vi "Benchmarks_DVR.vi"() -> ()   [LabVIEW 2024]
uses:
  <vilib>/numeric/Random Number (Range) U64.vi
  <vilib>/numeric/sub_Random U32.vi
panel:
  out "Waveform Chart":dbl(graph)
  out "Numeric":dbl
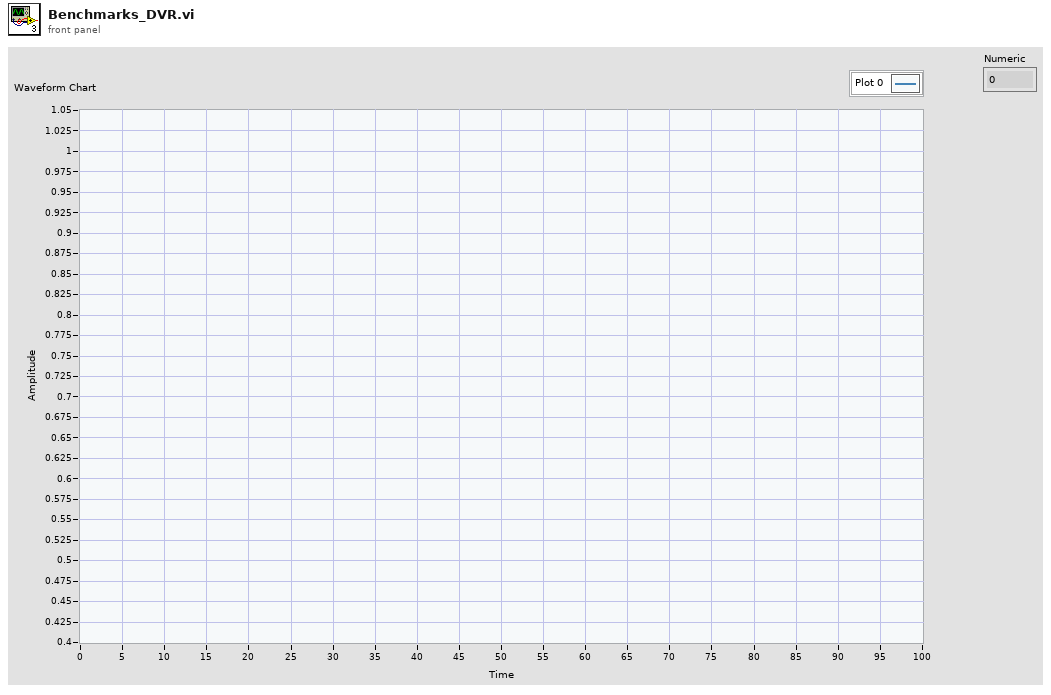
[diagram p1: front panel]
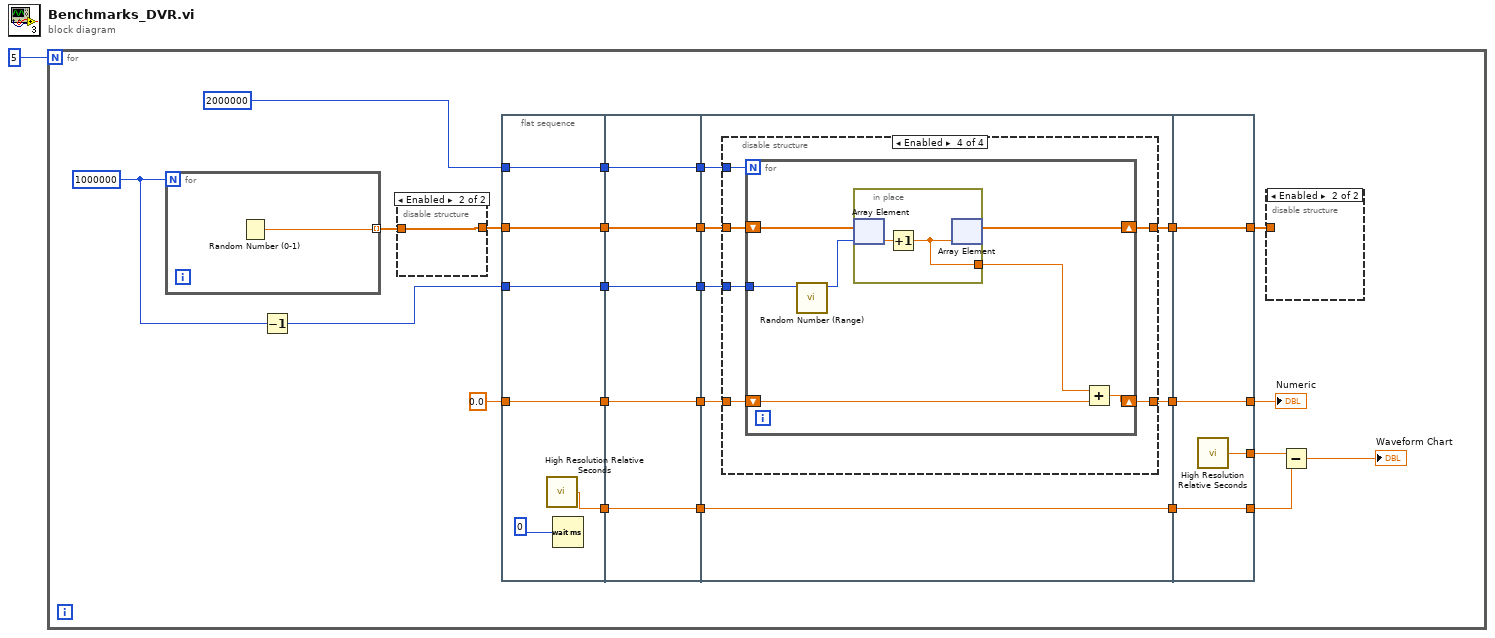
[diagram p0: block diagram]
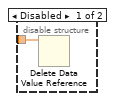
[diagram p2: hidden frame]
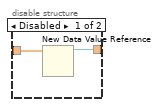
[diagram p3: hidden frame]
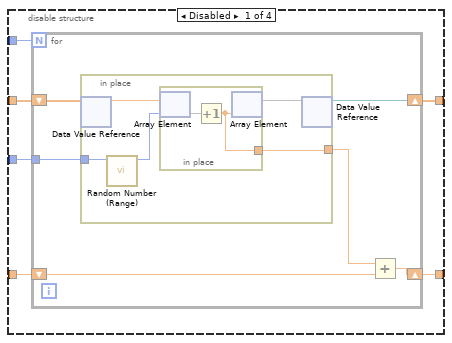
[diagram p4: hidden frame]
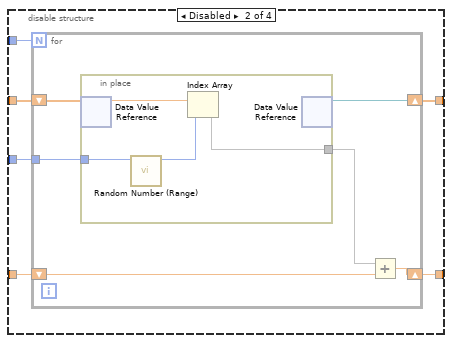
[diagram p5: hidden frame]
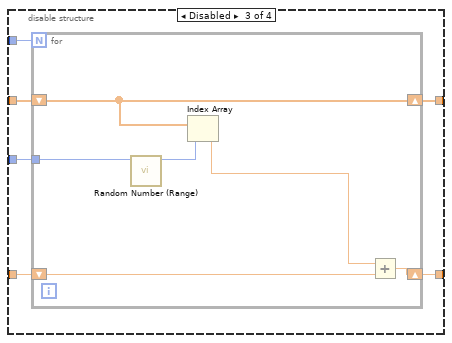
[diagram p6: hidden frame]
diagram:
  n1 = for {
    N: 5 -> [_]
    w10 = 1000000
    n2 = for {
      N: w10 -> [_]
      tunnel: [w114] -> w12 mode=indexing
      n3 = Random Number (0-1)() -> (number: 0 to 1=w114:dbl)
    }
    n4 = Decrement(x=w10) -> (x-1=w9:i32)
    n5 = disable-structure shown="Enabled" {
      disable-tunnel: w12 -> [w28 w29]
      disable-tunnel: [w27 w29] -> w11
      frame Disabled {
        n6 = New Data Value Reference(data value=w28) -> (data value reference=w27:refnum<data-value>)  [unwired: 1 in, 1 out]
      }
      frame Enabled {
      }
    }
    n7 = flat-sequence {
      tunnel: 2000000 -> [w32]
      tunnel: 0.0 -> [w33]
      tunnel: w9 -> [w34]
      tunnel: w11 -> [w35]
      tunnel: [w35] -> w25
      tunnel: [w34] -> w24
      tunnel: [w33] -> w23
      tunnel: [w32] -> w22
      tunnel: [w30] -> w21
      tunnel: [w40] -> w20
      tunnel: [w39] -> w19
      tunnel: [w38] -> w18
      tunnel: [w37] -> w17
      tunnel: w25 -> [w40]
      tunnel: w24 -> [w39]
      tunnel: w23 -> [w38]
      tunnel: w22 -> [w37]
      tunnel: w21 -> [w36]
      tunnel: [w36] -> w16
      tunnel: w20 -> [w47]
      tunnel: w19 -> [w46]
      tunnel: w18 -> [w45]
      tunnel: w17 -> [w42]
      tunnel: [w44] -> w15
      tunnel: [w43] -> w14
      tunnel: w16 -> [w41]
      tunnel: [w41] -> w13
      tunnel: [w112] -> w6
      tunnel: [w113] -> w7
      tunnel: w15 -> [w113]
      tunnel: w14 -> [w112]
      tunnel: [w111] -> w4
      tunnel: w13 -> [w110]
      tunnel: [w110] -> w3
      frame #0 {
        n8 = call <vilib>:"High Resolution Relative Seconds.vi"() -> ("relative seconds"=w30:dbl)
        n9 = Wait (ms)(milliseconds to wait=u32 0) -> ()  [unwired: 1 out]
      }
      frame #1 {
      }
      frame #2 {
        n10 = disable-structure shown="Enabled" {
          disable-tunnel: w47 -> [w53 w72 w88 w100]
          disable-tunnel: w46 -> [w52 w71 w87 w99]
          disable-tunnel: w45 -> [w51 w70 w86 w98]
          disable-tunnel: [w50 w69 w85 w97] -> w44
          disable-tunnel: [w49 w68 w84 w96] -> w43
          disable-tunnel: w42 -> [w48 w67 w83 w95]
          frame Disabled {
            n11 = for {
              N: w48 -> [_]
              tunnel: w52 -> [w58]
              shift-right: [w56] -> w50
              shift-left: w51 -> [w57]
              shift-right: [w54] -> w49
              shift-left: w53 -> [w59]
              n12 = in-place {
                in-place-border: w58 -> [w64]
                in-place-border: [w60] -> w55
                n13 = in-place-dvr #1(w59) -> (w63:dbl)  [unwired: 1 out]
                n14 = call-poly <vilib>:"Random Number (Range).vi"("upper bound (100)"=w64) -> ("number"=w62:u64)  [unwired: 10 in]
                n15 = in-place {
                  in-place-border: [w65] -> w60
                  n16 = in-place-array #2(w63, w62) -> (w66)
                  n17 = Increment(x=w66) -> (x+1=w65:dbl)
                  n18 = in-place-array #2(w65) -> (w61)  [unwired: 1 out]
                }
                n19 = in-place-dvr #1(w61) -> (w54:refnum<data-value>)  [unwired: 1 out]
              }
              n20 = Add(x=w55, y=w57) -> (x+y=w56:dbl)
            }
          }
          frame Disabled {
            n21 = for {
              N: w67 -> [_]
              tunnel: w71 -> [w77]
              shift-right: [w75] -> w69
              shift-left: w70 -> [w76]
              shift-right: [w73] -> w68
              shift-left: w72 -> [w78]
              n22 = in-place {
                in-place-border: w77 -> [w80]
                in-place-border: [w79] -> w74
                n23 = in-place-dvr #3(w78) -> (w82:dbl)  [unwired: 1 out]
                n24 = call-poly <vilib>:"Random Number (Range).vi"("upper bound (100)"=w80) -> ("number"=w81:u64)  [unwired: 10 in]
                n25 = Index Array(array=w82, index=w81) -> (element=w79)
                n26 = in-place-dvr #3() -> (w73:refnum<data-value>)  [unwired: 1 in, 1 out]
              }
              n27 = Add(x=w74, y=w76) -> (x+y=w75:dbl)
            }
          }
          frame Disabled {
            n28 = for {
              N: w83 -> [_]
              tunnel: w87 -> [w94]
              shift-right: [w92] -> w85
              shift-left: w86 -> [w93]
              shift-right: [w89] -> w84
              shift-left: w88 -> [w89]
              n29 = call-poly <vilib>:"Random Number (Range).vi"("upper bound (100)"=w94) -> ("number"=w90:u64)  [unwired: 10 in]
              n30 = Index Array(array=w89, index=w90) -> (element=w91:dbl)
              n31 = Add(x=w91, y=w93) -> (x+y=w92:dbl)
            }
          }
          frame Enabled {
            n32 = for {
              N: w95 -> [_]
              tunnel: w99 -> [w107]
              shift-right: [w105] -> w97
              shift-left: w98 -> [w106]
              shift-right: [w102] -> w96
              shift-left: w100 -> [w104]
              n33 = call-poly <vilib>:"Random Number (Range).vi"("upper bound (100)"=w107) -> ("number"=w103:u64)  [unwired: 10 in]
              n34 = in-place {
                in-place-border: [w108] -> w101
                n35 = in-place-array #4(w104, w103) -> (w109:dbl)
                n36 = Increment(x=w109) -> (x+1=w108:dbl)
                n37 = in-place-array #4(w108) -> (w102:dbl[])  [unwired: 1 out]
              }
              n38 = Add(x=w101, y=w106) -> (x+y=w105:dbl)
            }
          }
        }
      }
      frame #3 {
        n39 = call <vilib>:"High Resolution Relative Seconds.vi"() -> ("relative seconds"=w111:dbl)
      }
    }
    n40 = disable-structure shown="Enabled" {
      disable-tunnel: w6 -> [w26 _]
      frame Disabled {
        n41 = Delete Data Value Reference(data value reference=w26) -> ()  [unwired: 1 in, 2 out]
      }
      frame Enabled {
      }
    }
    n42 = Subtract(x=w4, y=w3) -> (x-y=→"Waveform Chart":dbl)
    "Numeric" <- w7
  }
